vi "String Trim Both Sides.vi"(10 "chars to trim":i32, 11 "string in":string) -> (3 "string out":string)   [LabVIEW 2014]
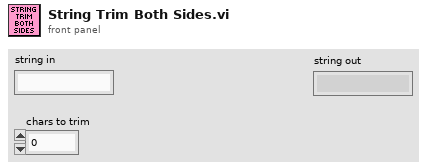
[diagram p1: front panel]
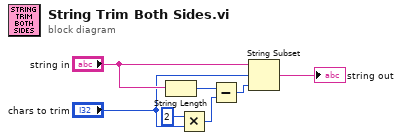
[diagram p0: block diagram]
diagram:
  n1 = String Length(string="string in") -> (length=w7:i32)
  n2 = Multiply(x=2, y="chars to trim") -> (x*y=w3:i32)
  n3 = Subtract(x=w7, y=w3) -> (x-y=w2:i32)
  n4 = String Subset(string="string in", offset (0)="chars to trim", length (rest)=w2) -> (substring=→"string out":string)
